vi "Test-All.vi"() -> ()   [LabVIEW 2023]
doc: "This VI implements the framework and scheduler for your robotics program. It should not be necessary to modify the framework. You are expected to add your code to the VIs called from Robot Main - the ones located in the Team Code folder within the project."
uses:
  Robot Global Data.vi
  <vilib>/Rock Robotics/WPI/ThirdParty/JAS_Junk/TrajLib/Trajectory_Library.lvlib
  <vilib>/Rock Robotics/WPI/DriverStation/WPI_DriverStationRobotMode2.ctl
panel:
  out "HighLimitSwitch":bool
  out "Low Limit Switch":bool
  out "HeightInch":dbl format="%9.1f"
  out "MotorOutDmd":dbl format="%9.2f"
  out "Robot Mode":T1
  in  "Finish":bool
  # "ELEVATOR"
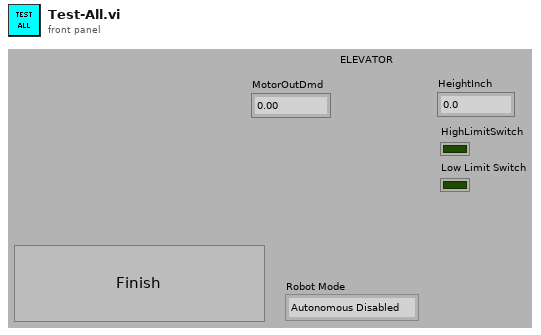
[diagram p1: front panel]
types:
  T1 = typedef "WPI_DriverStationRobotMode2.ctl" = enum16{"Autonomous Disabled", "Autonomous Enabled", "Teleop Disabled", "Teleop Enabled", "Disconnected", "Finish", "Test Disabled", "Test Enabled", "Emergency Stopped"}
  T2 = typedef "WPI_DriverStationMatch Info.ctl" = cluster{"Autonomous Elapsed Seconds":dbl, "TeleOp Elapsed Seconds":dbl, "Disabled Elapsed Seconds":dbl, "Visited Autonomous":bool, "Visited TeleOp":bool, "Visited Disabled":bool, "Autonomous Settings":cluster{"Autonomous Style":enum16{"Iterative", "Independent"}, "VI Refnum":refnum<vi>}}
  T3 = typedef "WPI_DriverStationDerivedRobotMode.ctl" = enum16{"Init", "Execute", "Stop"}
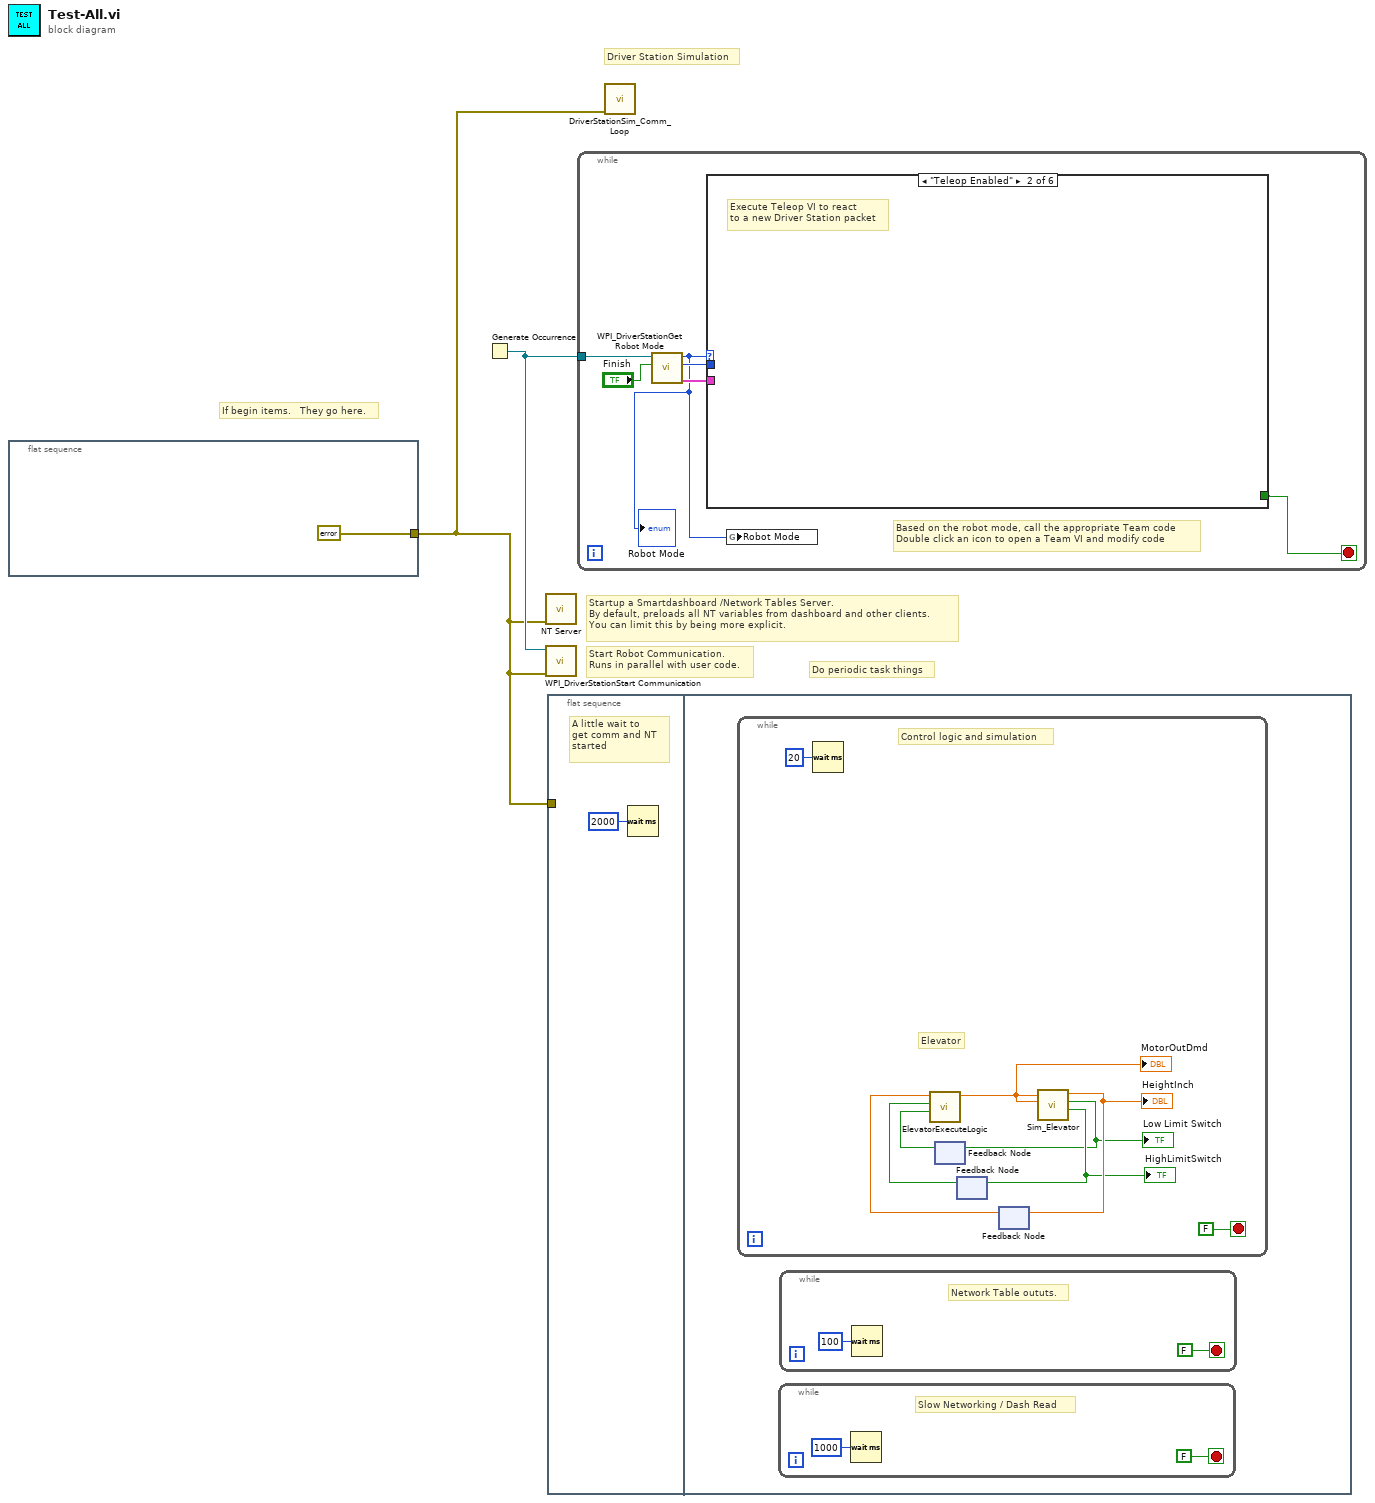
[diagram p0: block diagram]
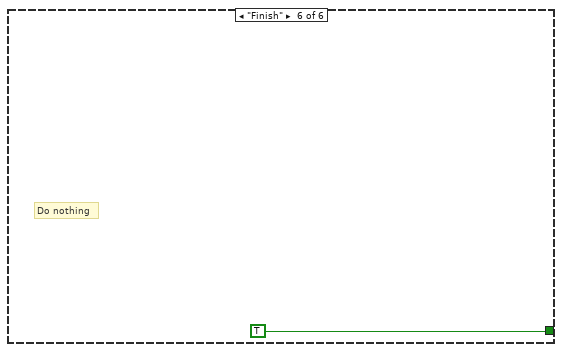
[diagram p6: hidden frame]
diagram:
  # "Driver Station Simulation"
  # "If begin items.   They go here."
  # "Do periodic task things"
  # "Startup a Smartdashboard /Network Tables Server.\nBy default, preloads all NT variables from dashboard and other clients.\nYou can limit this by being more explicit."
  # "Start Robot Communication.\nRuns in parallel with user code."
  n1 = flat-sequence {
    tunnel: [errorcluster {"status"=FALSE, "code"=0, "source"=""} ("error in (no error)")] -> w1
    frame #0 {
    }
  }
  n2 = Generate Occurrence() -> (w2:refnum<k4>)
  n3 = call <vilib>:"NT Server.vi"("error in (no error)"=w1) -> ()  [unwired: 10 in, 1 out]
  n4 = call <vilib>:"WPI_DriverStationStart Communication.vi"("error in (no error)"=w1, "occurrence"=w2) -> ()  [unwired: 1 in, 9 out]
  n5 = flat-sequence {
    tunnel: w1 -> [_]
    frame #0 {
      # "A little wait to\nget comm and NT\nstarted"
      n6 = Wait (ms)(milliseconds to wait=u32 2000) -> ()  [unwired: 1 out]
    }
    frame #1 {
      n7 = while {
        stop <- FALSE stop-if-true
        # "Elevator"
        # "Control logic and simulation"
        n8 = Wait (ms)(milliseconds to wait=u32 20) -> ()  [unwired: 1 out]
        n9 = feedback #1() -> (w10:bool)  [unwired: 1 in]
        n10 = feedback #2() -> (w12:bool)  [unwired: 1 in]
        n11 = feedback #3() -> (w14:dbl)  [unwired: 1 in]
        n12 = call "ElevatorExecuteLogic.vi"("LowLimitSwitch"=w10, "HighLimitSwitch"=w12, "PositionHeight"=w14) -> ("MotorDemand"=w9:dbl)  [unwired: 7 in, 1 out]
        "MotorOutDmd" <- w9
        n13 = call "Sim_Elevator.vi"("Motor2 Dmd"=w9, "Motor1 Dmd"=w9) -> ("HighLimitSwitch"=w13:bool, "Low Limit Switch"=w11:bool, "ElevHeightInch"=w15:dbl)  [unwired: 7 in]
        "HeightInch" <- w15
        "Low Limit Switch" <- w11
        "HighLimitSwitch" <- w13
        n14 = feedback-in #1(w11) -> ()
        n15 = feedback-in #2(w13) -> ()
        n16 = feedback-in #3(w15) -> ()
      }
      n17 = while {
        stop <- FALSE stop-if-true
        # "Slow Networking / Dash Read"
        n18 = Wait (ms)(milliseconds to wait=u32 1000) -> ()  [unwired: 1 out]
      }
      n19 = while {
        stop <- FALSE stop-if-true
        # "Network Table oututs."
        n20 = Wait (ms)(milliseconds to wait=u32 100) -> ()  [unwired: 1 out]
      }
    }
  }
  n21 = while {
    tunnel: w2 -> [w23]
    stop <- w18 stop-if-true
    # "Based on the robot mode, call the appropriate Team code\nDouble click an icon to open a Team VI and modify code"
    n22 = call <vilib>:"WPI_DriverStationGet Robot Mode.vi"("Finish"="Finish", "DS Occurrence"=w23) -> ("Match Info out"=w20:T2, "Call Context"=w22:T3, "Robot Mode"=w19:T1)  [unwired: 7 out]
    "Robot Mode" <- w19
    n23 = case shown="\"Teleop Enabled\"" w19 {
      tunnel: w22 -> [_ _ _ _ _ _]
      tunnel: w20 -> [_ _ _ _ _ _]
      tunnel: [_ _ _ _ _ TRUE] -> w18
      frame "Autonomous Enabled" {
        # "Do nothing...."
      }
      frame "Teleop Enabled" {
        # "Execute Teleop VI to react\nto a new Driver Station packet"
      }
      frame "Test Disabled", "Test Enabled" {
        # "Do nothing"
      }
      frame "Autonomous Disabled", "Teleop Disabled" {
        # "Do nothing."
      }
      frame "Disconnected", Default {
        # "Driver Station packet didn't arrive.\nPossibly useful for diagnostics"
      }
      frame "Finish" {
        # "Do nothing"
      }
    }
    n24 = global write "Robot Global Data.vi" "Robot Mode"(w19) -> ()
  }
  n25 = call <vilib>:"DriverStationSim_Comm_Loop.vi"("error in (no error)"=w1) -> ()  [unwired: 11 in]
